vi "CommonVIs_TypeDescNonNameDepentent.vi"(0 "Type DescriptorNameDependent":i16[](array[numeric]), 1 "LabelText":string) -> (14 "Type DescriptorNonNameDependent":i16[](array[numeric]) format="%.0x")   [LabVIEW 2020]
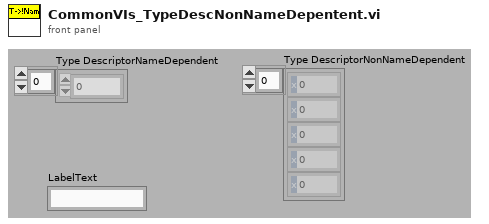
[diagram p1: front panel]
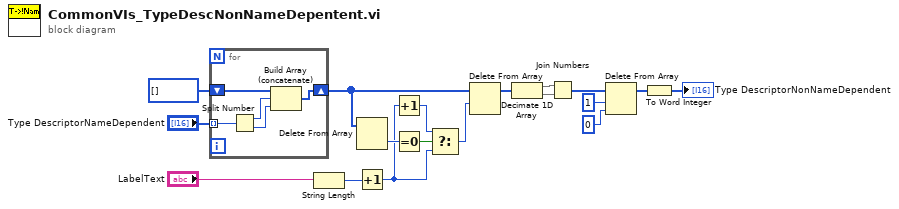
[diagram p0: block diagram]
diagram:
  n1 = for {
    tunnel: "Type DescriptorNameDependent" -> [w23] mode=indexing
    shift-right: [w21] -> w16
    shift-left: u8[] [] -> [w22]
    n2 = Split Number(x=w23) -> (hi(x)=w20:u8, lo(x)=w19:u8)
    n3 = Build Array (concatenate)(w22, w20, w19) -> (w21:u8[])
  }
  n4 = String Length(string="LabelText") -> (length=w6:i32)
  n5 = Delete From Array(array=w16) -> (deleted portion=w15:u8)  [unwired: 2 in, 1 out]
  n6 = Increment(x=w6) -> (x+1=w13:i32)
  n7 = Increment(x=w13) -> (x+1=w12:i32)
  n8 = Equal To 0?(x=w15) -> (x = 0?=w14:bool)
  n9 = Select(t=w12, s=w14, f=w13) -> (s? t:f=w11:i32)
  n10 = Delete From Array(array=w16, length=w11) -> (array with subset deleted=w8:u8[])  [unwired: 1 in, 1 out]
  n11 = Decimate 1D Array(w8) -> (w10:u8[], w9:u8[])
  n12 = Join Numbers(hi=w10, lo=w9) -> ((hi.lo)=w5:u16[])
  n13 = Delete From Array(array=w5, length=1, index=0) -> (array with subset deleted=w2:u16[])  [unwired: 1 out]
  n14 = To Word Integer(number=w2) -> (16bit integer=→"Type DescriptorNonNameDependent":i16[])
